vi "Write Serial Num.vi"(8 "error in (no error)":errorcluster, 10 "Serial Num":string, 11 "Alicat in":refnum<class "Alicat.lvclass">) -> (0 "error out":errorcluster, 3 "Alicat out":refnum<class "Alicat.lvclass">)   [LabVIEW 2014, in "Alicat.lvlib" / "Alicat.lvclass"]
uses:
  Alicat.lvclass
  Alicat.lvclass/Alicat.ctl
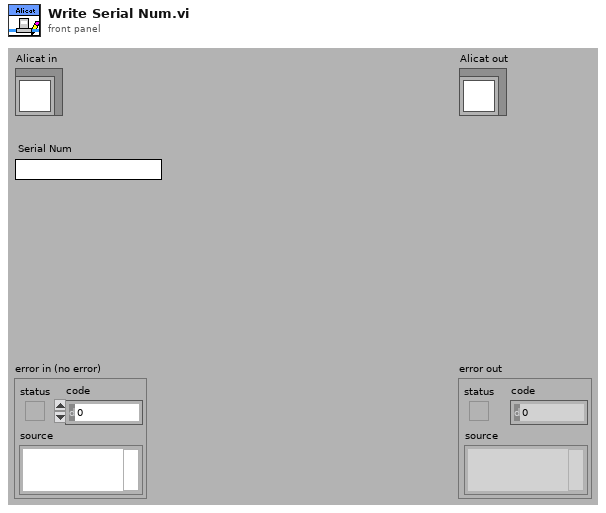
[diagram p1: front panel]
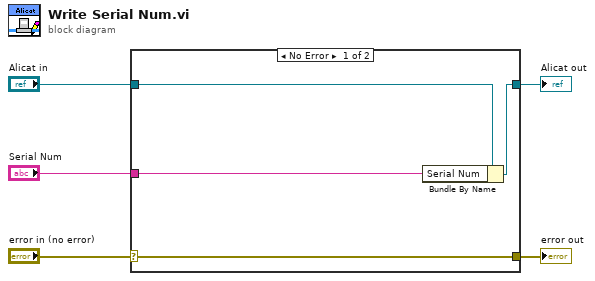
[diagram p0: block diagram]
diagram:
  n1 = case shown="No Error" "error in (no error)" {
    selector: "error in (no error)" -> [w9 w10]
    tunnel: [w9 w10] -> w4
    tunnel: [w7 w11] -> w2
    tunnel: "Alicat in" -> [w8 w11]
    tunnel: "Serial Num" -> [w6 _]
    frame No Error {
      n2 = Bundle By Name(cluster=w8, "Serial Num"=w6) -> (w7:refnum<class "Alicat.lvclass">)
    }
    frame Error {
    }
  }
  "error out" <- w4
  "Alicat out" <- w2
